vi "Swap Panel Down.vi"(8 "error in (no error)":errorcluster, 10 "Panel":refnum<class "Panel.lvclass">, 11 "PanelArray in":refnum<class "PanelArray.lvclass">) -> (0 "error out":errorcluster, 3 "PanelArray out":refnum<class "PanelArray.lvclass">)   [LabVIEW 2018, in "OOPanel.lvlib" / "PanelArray.lvclass"]
uses:
  PanelArray.lvclass
  Panel/Panel.lvclass
  PanelArray.lvclass/PanelArray.ctl
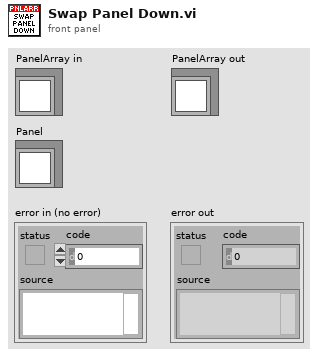
[diagram p1: front panel]
types:
  T1 = typedef "OOPanel.lvlib/PanelArray.lvclass/Ref Data.ctl" = cluster{"State":T2, "Refs":T3, "Events":T4, "Scrolling":T5, "Panels":T6}
  T2 = typedef "OOPanel.lvlib/PanelArray.lvclass/State.ctl" = cluster{"Defer Updates":bool, "Running":bool, "Dynamic Sizing":bool, "Borders":bool}
  T3 = typedef "OOPanel.lvlib/PanelArray.lvclass/Refs.ctl" = cluster{"SubPanels":refnum<vi>[], "Scrollbar":refnum<vi>, "Owning Panel":refnum<vi>}
  T4 = typedef "OOPanel.lvlib/PanelArray.lvclass/Events.ctl" = cluster{"Close":refnum<user-event>}
  T5 = typedef "OOPanel.lvlib/PanelArray.lvclass/Scrolling.ctl" = cluster{"Size":i32, "Max":i32, "Current":i32, "Top Index":i32, "Heights":i32[]}
  T6 = typedef "OOPanel.lvlib/PanelArray.lvclass/Panels.ctl" = cluster{"All":refnum<class "Panel.lvclass">[], "Visible":refnum<class "Panel.lvclass">[], "Blank":refnum<class "ArrayBlank.lvclass">}
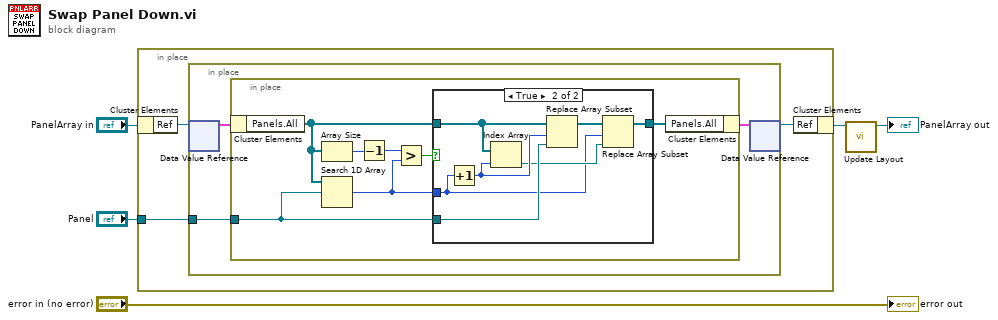
[diagram p0: block diagram]
diagram:
  n1 = in-place {
    in-place-border: "Panel" -> [w8]
    n2 = in-place-cluster #1("PanelArray in") -> ("Ref"=w7:refnum<data-value>)
    n3 = in-place {
      in-place-border: w8 -> [w9]
      n4 = in-place-dvr #2(w7) -> (w11:T1)  [unwired: 1 out]
      n5 = in-place {
        in-place-border: w9 -> [w17]
        n6 = in-place-cluster #3(w11) -> ("Panels.All"=w16:refnum<class "Panel.lvclass">[])
        n7 = Array Size(array=w16) -> (size(s)=w15:i32)
        n8 = Search 1D Array(1D array=w16, element=w17) -> (index of element=w13:i32)  [unwired: 1 in]
        n9 = Decrement(x=w15) -> (x-1=w14:i32)
        n10 = Greater?(x=w14, y=w13) -> (0:w12:bool)
        n11 = case shown="True" w12 {
          tunnel: w13 -> [_ w21]
          tunnel: w16 -> [w19 w26]
          tunnel: [w19 w20] -> w18
          tunnel: w17 -> [_ w25]
          frame False {
          }
          frame True {
            n12 = Increment(x=w21) -> (x+1=w24:i32)
            n13 = Index Array(array=w26, index=w24) -> (element=w22:refnum<class "Panel.lvclass">)
            n14 = Replace Array Subset(array=w26, new element=w25, index=w24) -> (w23:refnum<class "Panel.lvclass">[])
            n15 = Replace Array Subset(array=w23, new element=w22, index=w21) -> (w20:refnum<class "Panel.lvclass">[])
          }
        }
        n16 = in-place-cluster #3("Panels.All"=w18) -> (w10:T1)
      }
      n17 = in-place-dvr #2(w10) -> (w6:refnum<data-value>)  [unwired: 1 out]
    }
    n18 = in-place-cluster #1("Ref"=w6) -> (w2:refnum<class "PanelArray.lvclass">)
  }
  n19 = call "Update Layout.vi"("PanelArray in"=w2) -> ("PanelArray out"=→"PanelArray out":refnum<class "PanelArray.lvclass">)  [unwired: 9 in, 1 out]
  "error out" <- "error in (no error)"
